vi "Convex Hull Graham Scan.vi"(2 "Center (Bottom Mid Point)":T3={"X"=-1, "Y"=-1}, 3 "Bounding Rectangle (Entire Array)":T2={"Left"=-1, "Top"=-1, "Right"=-1, "Bottom"=-1}, 4 "Plane":bool[][](array[boolean])) -> (0 "Interior Points":T1[](array[typedef]), 1 "Convex Hull":T1[](array[typedef]))   [LabVIEW 2018]
uses:
  Graham Scan Origin Point STYP.ctl
  Graham Scan Bounding Rectangle STYP.ctl
  Graham Scan Point.ctl
  eaf5b3b9-2e87-43fa-90dc-088ca0f29dd0.vi
  d67e6263-d603-42e7-bf5e-babf5bc42cce.vi
  523a4078-f151-4d85-8003-425d013a5b44.vi
  d75970e5-f0a1-4c50-87ac-54c35781b05a.vi
  fd4f598d-7994-474b-93f9-4ac3989735a0.vi
  a06fee5f-fd5c-4d2f-95bd-33159e0feda1.vi
  d157a3a7-1922-4b04-a71b-69ebc794f7ed.vi
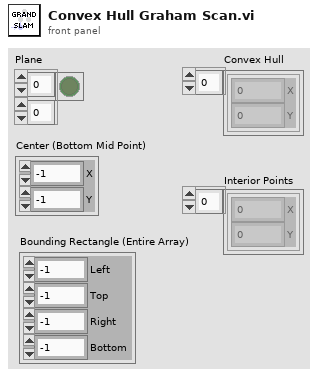
[diagram p1: front panel]
types:
  T1 = typedef "Graham Scan Point.ctl" = cluster{"X":i32, "Y":i32}
  T2 = typedef "Graham Scan Bounding Rectangle STYP.ctl" = cluster{"Left":i32, "Top":i32, "Right":i32, "Bottom":i32}
  T3 = typedef "Graham Scan Origin Point STYP.ctl" = cluster{"X":i32, "Y":i32}
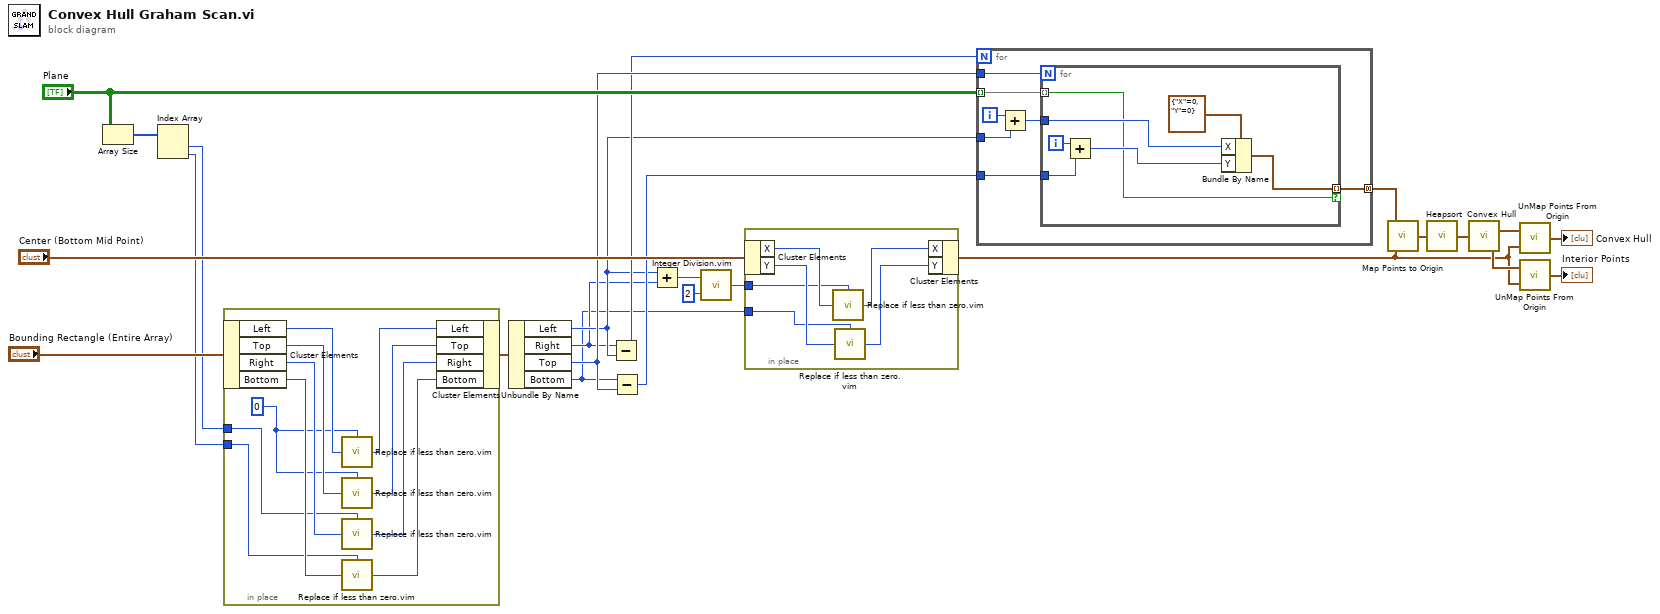
[diagram p0: block diagram]
diagram:
  n1 = Array Size(array="Plane") -> (size(s)=w24:i32[])
  n2 = Index Array(array=w24) -> (element #1=w21:i32, element #2=w15:i32)  [unwired: 2 in]
  n3 = in-place {
    in-place-border: w21 -> [w30]
    in-place-border: w15 -> [w29]
    w31 = 0
    n4 = in-place-cluster #1("Bounding Rectangle (Entire Array)") -> ("Left"=w35:i32, "Top"=w34:i32, "Right"=w33:i32, "Bottom"=w32:i32)
    n5 = call "Replace if less than zero.vim"("Replacement (0)"=w31, "X"=w35) -> ("Y"=w28:i32)  [unwired: 2 in]
    n6 = call "Replace if less than zero.vim"("Replacement (0)"=w31, "X"=w34) -> ("Y"=w27:i32)  [unwired: 2 in]
    n7 = call "Replace if less than zero.vim"("Replacement (0)"=w30, "X"=w33) -> ("Y"=w26:i32)  [unwired: 2 in]
    n8 = call "Replace if less than zero.vim"("Replacement (0)"=w29, "X"=w32) -> ("Y"=w25:i32)  [unwired: 2 in]
    n9 = in-place-cluster #1("Left"=w28, "Top"=w27, "Right"=w26, "Bottom"=w25) -> (w19:T2)
  }
  n10 = Unbundle By Name(w19) -> ("Left"=w12:i32, "Right"=w11:i32, "Top"=w18:i32, "Bottom"=w8:i32)
  n11 = Subtract(x=w11, y=w12) -> (x-y=w14:i32)
  n12 = Subtract(x=w8, y=w18) -> (x-y=w17:i32)
  n13 = Add(x=w12, y=w11) -> (x+y=w10:i32)
  n14 = call "Integer Division.vim"("Y"=2, "X"=w10) -> ("X // Y"=w9:i32)
  n15 = in-place {
    in-place-border: w9 -> [w37]
    in-place-border: w8 -> [w36]
    n16 = in-place-cluster #2("Center (Bottom Mid Point)") -> ("X"=w41:i32, "Y"=w40:i32)
    n17 = call "Replace if less than zero.vim"("Replacement (0)"=w37, "X"=w41) -> ("Y"=w39:i32)  [unwired: 2 in]
    n18 = call "Replace if less than zero.vim"("Replacement (0)"=w36, "X"=w40) -> ("Y"=w38:i32)  [unwired: 2 in]
    n19 = in-place-cluster #2("X"=w39, "Y"=w38) -> (w3:T3)
  }
  n20 = for {
    N: w14 -> [_]
    tunnel: "Plane" -> [w46] mode=indexing
    tunnel: w12 -> [w47]
    tunnel: w18 -> [w45]
    tunnel: w17 -> [w44]
    tunnel: [w42] -> w16 mode=concatenating
    i -> [w48]
    n21 = Add(x=w48, y=w47) -> (x+y=w43:i32)
    n22 = for {
      N: w45 -> [_]
      tunnel: w46 -> [w49] mode=indexing
      tunnel: w44 -> [w54]
      tunnel: w43 -> [w52]
      tunnel: [w50] -> w42 mode=indexing if=w49
      i -> [w55]
      n23 = Add(x=w55, y=w54) -> (x+y=w51:i32)
      n24 = Bundle By Name(cluster=T1 {"X"=0, "Y"=0} ("Point"), "X"=w52, "Y"=w51) -> (w50:T1)
    }
  }
  n25 = call "Map Points to Origin.vi"("New Origin"=w3, "Points"=w16) -> ("Mapped Points"=w7:T1[])
  n26 = call "Heapsort.vi"("Array"=w7) -> ("Sorted Array"=w6:T1[])
  n27 = call "Convex Hull.vi"("Sorted Array"=w6) -> ("Interior Points"=w4:T1[], "Convex Hull"=w5:T1[])  [unwired: 2 in]
  n28 = call "UnMap Points From Origin.vi"("New Origin"=w3, "Points"=w5) -> ("Mapped Points"=→"Convex Hull":T1[])
  n29 = call "UnMap Points From Origin.vi"("New Origin"=w3, "Points"=w4) -> ("Mapped Points"=→"Interior Points":T1[])
